vi "FPGA SPI_Globals.vi"() -> ()   [LabVIEW 2011]
uses:
  Controls/FPGA SPI_Cmd.ctl
panel:
  in  "SPI_Cmd":T1=enum."Configure"
  in  "SPI_Clock Divider":u32=20
  in  "SPI_CS Active State":bool caption="SPI_CS \nActive State"
  in  "SPI_CPOL":bool
  in  "SPI_CPHA":bool
  in  "SPI_CS":u8=128 format="%08b"
  in  "SPI_Total Bits":u16=8
  in  "SPI_Total Bytes":u16=1
  out "SPI_Done":bool
  out "SPI_Start":bool
  in  "SPI_Port":u8
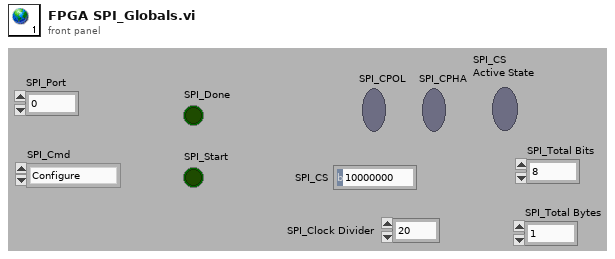
[diagram p1: front panel]
types:
  T1 = typedef "FPGA SPI_Cmd.ctl" = enum8{"Idle", "Write/Read SPI", "Configure"}
diagram:
